vi "execute.vi"(8 "error in (no error)":errorcluster, 10 "Context in":refnum<class "Context.lvclass">, 11 "LowerM1M3Command in":refnum<class "LowerM1M3Command.lvclass">) -> (0 "error out":errorcluster, 2 "Context out":refnum<class "Context.lvclass">, 3 "LowerM1M3Command out":refnum<class "LowerM1M3Command.lvclass">)   [LabVIEW 2016, in "LowerM1M3Command.lvclass"]
uses:
  LowerM1M3Command.lvclass
  Context/Context.lvclass
  LowerM1M3Command.lvclass/LowerM1M3Command.ctl
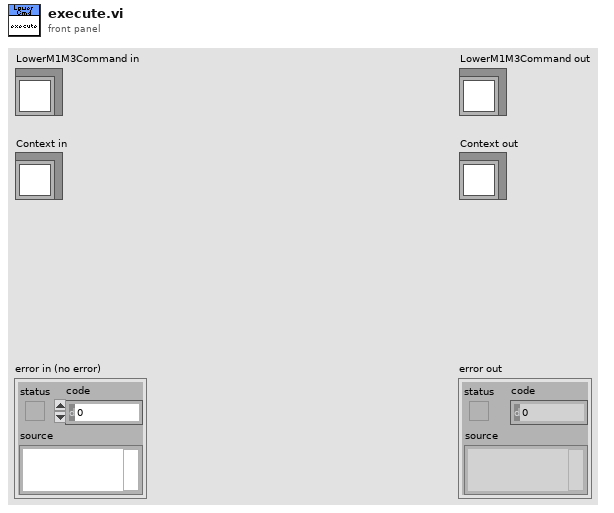
[diagram p1: front panel]
types:
  T1 = typedef "M1M3SupportTopics.lvlib/CommandLowerM1M3.ctl" = cluster{"CommandId":T2, "LowerM1M3":bool}
  T2 = typedef "M1M3SupportTopics.lvlib/CommandId.ctl" = i32
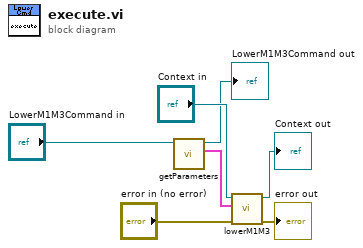
[diagram p0: block diagram]
diagram:
  n1 = call "getParameters.vi"("LowerM1M3Command in"="LowerM1M3Command in") -> ("Parameters"=w3:T1, "LowerM1M3Command out"=→"LowerM1M3Command out":refnum<class "LowerM1M3Command.lvclass">)  [unwired: 9 in]
  n2 = call-dynamic "lowerM1M3.vi"("error in (no error)"="error in (no error)", "Parameters"=w3, "Context in"="Context in") -> ("error out"=→"error out":errorcluster, "Context out"=→"Context out":refnum<class "Context.lvclass">)  [unwired: 7 in]
